vi "Unbundle Enabled Hardware Control.vi"(11 "Control in":refnum<vi>) -> (0 "data out":T1, 1 "Enabled and not yet connected":bool, 2 "Device":string, 3 "Control out":refnum<vi>)   [LabVIEW 2020]
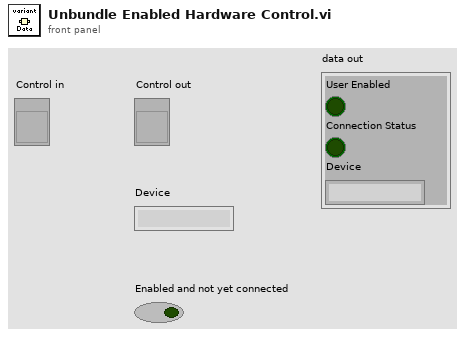
[diagram p1: front panel]
types:
  T1 = cluster{"User Enabled":bool, "Connection Status":bool, "Device":string}
  T2 = cluster{"Enable":bool, "Status":bool, "Device":string}
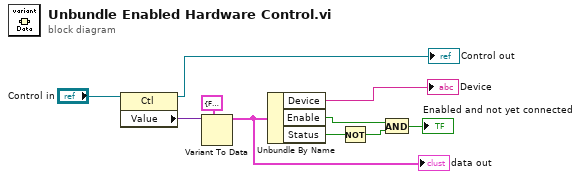
[diagram p0: block diagram]
diagram:
  n1 = property class="Ctl"(reference="Control in") -> (reference out=→"Control out":refnum<vi>, "Value"=w2:variant)  [unwired: 1 in, 1 out]
  n2 = Variant To Data(type=T2 {"Enable"=FALSE, "Status"=FALSE, "Device"=""} ("Device"), Variant=w2) -> (data=w4:T2)  [unwired: 1 in, 1 out]
  "data out" <- w4
  n3 = Unbundle By Name(w4) -> ("Device"=→"Device":string, "Enable"=w9:bool, "Status"=w7:bool)
  n4 = Not(x=w7) -> (.not. x?=w8:bool)
  n5 = And(x=w9, y=w8) -> (x .and. y?=→"Enabled and not yet connected":bool)
